vi "CanReceivePass.vi"(8 "error in (no error)":errorcluster, 9 "GameRef":refnum<data-value>, 10 "Robot":refnum<class "Robot.lvclass">, 11 "object in":refnum<class "SupportAttackerRole.lvclass">) -> (0 "error out":errorcluster, 2 "CanReceivePass":bool=TRUE, 3 "object out":refnum<class "SupportAttackerRole.lvclass">)   [LabVIEW 2023, in "SupportAttackerRole.lvclass"]
uses:
  SupportAttackerRole.lvclass
  Robot_class/Robot.lvclass
  C:/Users/ebert/Documents/codes/SSL/repo/SSL_AI/Object_class/Object.lvclass
  Game_class/Game.lvclass
  Game_class/Game.lvclass/Game.ctl
  Object_class/Object.lvclass/Object.ctl
  <vilib>/Analysis/_algsub.llb/Real Vector Norm.vi
  Game_class/Read BallRef.vi
  Object_class/Read position(x,y).vi
  Ball_class/Ball.lvclass
  Zone_class/Zone.lvclass
  Utilities_class/Utilities.lvclass
  <vilib>/Analysis/NI_AALPro.lvlib
panel:
  in  "threshold":dbl
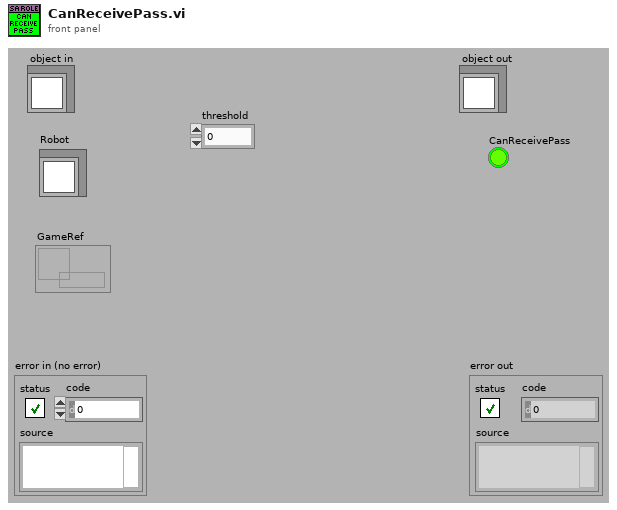
[diagram p1: front panel]
types:
  T1 = typedef "STPParameters.ctl" = cluster{"Skills":T2, "TestSkill":T4, "Events":cluster{"distanceToBallPossession":dbl, "timeForPossessionThreshold":dbl}, "Criteria":cluster{"OpenAngleToGoal":cluster{"minAngle":dbl, "maxAngle":dbl, "minEvaluation":dbl}, "PassDistance":cluster{"maxDistance":dbl, "minDistance":dbl}, "ShotInterception":cluster{"shotSpeed":dbl, "minEnemySpeed":dbl, "minEvaluation":dbl, "maxEnemySpeed":dbl}, "OneTouchShot":cluster{"MaxAngle":dbl, "minEvaluation":dbl}, "PassInterception":cluster{"minEnemySpeed":dbl, "maxEnemySpeed":dbl, "chipPassDistance":dbl, "chipPassEval":dbl, "minEvaluation":dbl}}, "minPassSpeed":dbl, "maxPassSpeed":dbl, "AllyTeamIds":T5[], "ReceiverSpeed":dbl, "minEvaluationToShoot":dbl}
  T2 = typedef "Skills.ctl" = cluster{"CirculateBall":T3, "ProtectBall":cluster{"DistanceFromBall":dbl}}
  T3 = typedef "CIrculateSkillParameters.ctl" = cluster{"rotationAngle":dbl, "velocityFactor":dbl, "OrientationFactor":dbl}
  T4 = typedef "TestSkills.ctl" = enum16{"AlignSkill", "PassSkill", "CirculateBall", "OneTouchShotSkill", "KickToSkill_v2", "ShootSkill", "InterceptBall", "Exit", "GoToSkill_v2"}
  T5 = typedef "AllyTeam.ctl" = enum16{"Keeper", "Defender", "Attacker"}
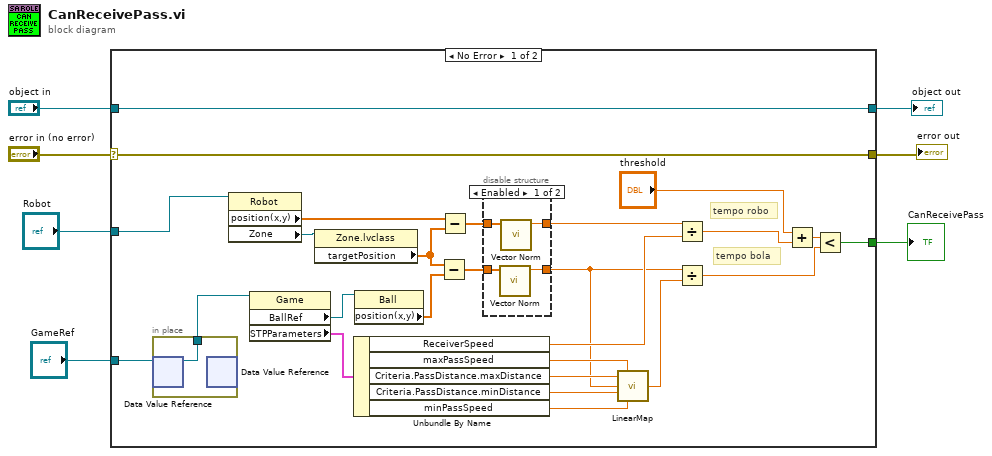
[diagram p0: block diagram]
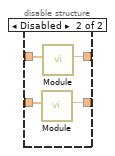
[diagram p2: hidden frame]
diagram:
  n1 = case shown="No Error" "error in (no error)" {
    selector: "error in (no error)" -> [w33 w44]
    tunnel: [w33 w44] -> w6
    tunnel: [w32 w43] -> w4
    tunnel: "object in" -> [w32 w43]
    tunnel: "Robot" -> [w31 _]
    tunnel: "GameRef" -> [w30 _]
    tunnel: [w9 _] -> w1
    frame No Error {
      # "tempo bola"
      # "tempo robo"
      n2 = in-place {
        in-place-border: [w42] -> w29
        n3 = in-place-dvr #1(w30) -> (w42:refnum<class "Game.lvclass">)  [unwired: 1 out]
        n4 = in-place-dvr #1() -> ()  [unwired: 1 in, 2 out]
      }
      n5 = property class="Robot"(reference=w31) -> ("position(x,y)"=w20:dbl[], "Zone"=w28:refnum<class "Zone.lvclass">)  [unwired: 1 in, 2 out]
      n6 = property class="Game"(reference=w29) -> ("BallRef"=w22:refnum<class "Ball.lvclass">, "STPParameters"=w23:T1)  [unwired: 1 in, 2 out]
      n7 = property class="Zone.lvclass"(reference=w28) -> ("targetPosition"=w19:dbl[])  [unwired: 1 in, 2 out]
      n8 = Unbundle By Name(w23) -> ("ReceiverSpeed"=w14:dbl, "maxPassSpeed"=w25:dbl, "Criteria.PassDistance.maxDistance"=w27:dbl, "Criteria.PassDistance.minDistance"=w26:dbl, "minPassSpeed"=w24:dbl)
      n9 = property class="Ball"(reference=w22) -> ("position(x,y)"=w21:dbl[])  [unwired: 1 in, 2 out]
      n10 = Subtract(x=w19, y=w21) -> (x-y=w17:dbl[])
      n11 = Subtract(x=w20, y=w19) -> (x-y=w18:dbl[])
      n12 = disable-structure shown="Enabled" {
        disable-tunnel: w18 -> [w37 w40]
        disable-tunnel: w17 -> [w36 w41]
        disable-tunnel: [w35 w39] -> w15
        disable-tunnel: [w34 w38] -> w13
        frame Enabled {
          n13 = call-poly <vilib>:"Vector Norm.vi"("Input Vector"=w36) -> ("norm"=w34:dbl)  [unwired: 9 in, 1 out]
          n14 = call-poly <vilib>:"Vector Norm.vi"("Input Vector"=w37) -> ("norm"=w35:dbl)  [unwired: 9 in, 1 out]
        }
        frame Disabled {
          n15 = call "Module.vi"("2D vector"=w41) -> ("Modulo"=w38:dbl)  [unwired: 8 in, 2 out]
          n16 = call "Module.vi"("2D vector"=w40) -> ("Modulo"=w39:dbl)  [unwired: 8 in, 2 out]
        }
      }
      n17 = call "LinearMap.vi"("MaxY"=w25, "MaxX"=w27, "X"=w13, "MinX"=w26, "MinY"=w24) -> ("Y"=w16:dbl)  [unwired: 8 in, 2 out]
      n18 = Divide(x=w15, y=w14) -> (x/y=w8:dbl)
      n19 = Divide(x=w13, y=w16) -> (x/y=w10:dbl)
      n20 = Add(x="threshold", y=w8) -> (x+y=w11:dbl)
      n21 = Less?(x=w11, y=w10) -> (x < y?=w9:bool)
    }
    frame Error {
    }
  }
  "error out" <- w6
  "object out" <- w4
  "CanReceivePass" <- w1
